vi "Module - Network Stream HMI.vi"(11 "Stop":bool) -> ()   [LabVIEW 2020]
uses:
  Control/State - NS HMI.ctl
  Control/State - eFGV.ctl
  Control/Section.ctl
  <vilib>/dex/Stream Element Allocation Mode.ctl
  <resource>/objmgr/ni.dex.rc
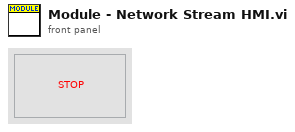
[diagram p1: front panel]
types:
  T1 = cluster{"T_Out":i32, "Event Ref":refnum<event-registration>, "NS Connected?":bool, "NS Endpoint":refnum<k21>, "Stop Main":bool, "NS Setting":cluster{"Timeout":i32, "Buffer Size":i32, "Ip Address":string, "Writer Name":string}}
  T2 = typedef "State - NS HMI.ctl" = enum16{"Init", "Register Event", "Read NS Setting", "Idle", "Create Reader Endpoint", "Check Connection Network Stream", "Read Stream Data", "Destroy NS", "Unregister Event", "Close"}
  T3 = typedef "State - eFGV.ctl" = enum16{"Init", "Read", "Write", "Exit"}
  T4 = enum16{"Timeout", "Buffer Size", "Ip Address", "Writer Name"}
  T5 = typedef "Section.ctl" = enum16{"Software Setup", "Config", "Setup", "Network Stream", "MQTT Client", "Setting", "Sample Interval", "Calibration", "Pre-Ranging", "Overrun", "Static", "Filter", "Properties", "Alarm", "Device", "Logging"}
  T6 = typedef "Stream Element Allocation Mode.ctl" = u32
  T7 = enum32{"invalid app kind", "Development System", "Run Time System", "Student Edition", "Embedded LabVIEW", "Evaluation", "Custom"}
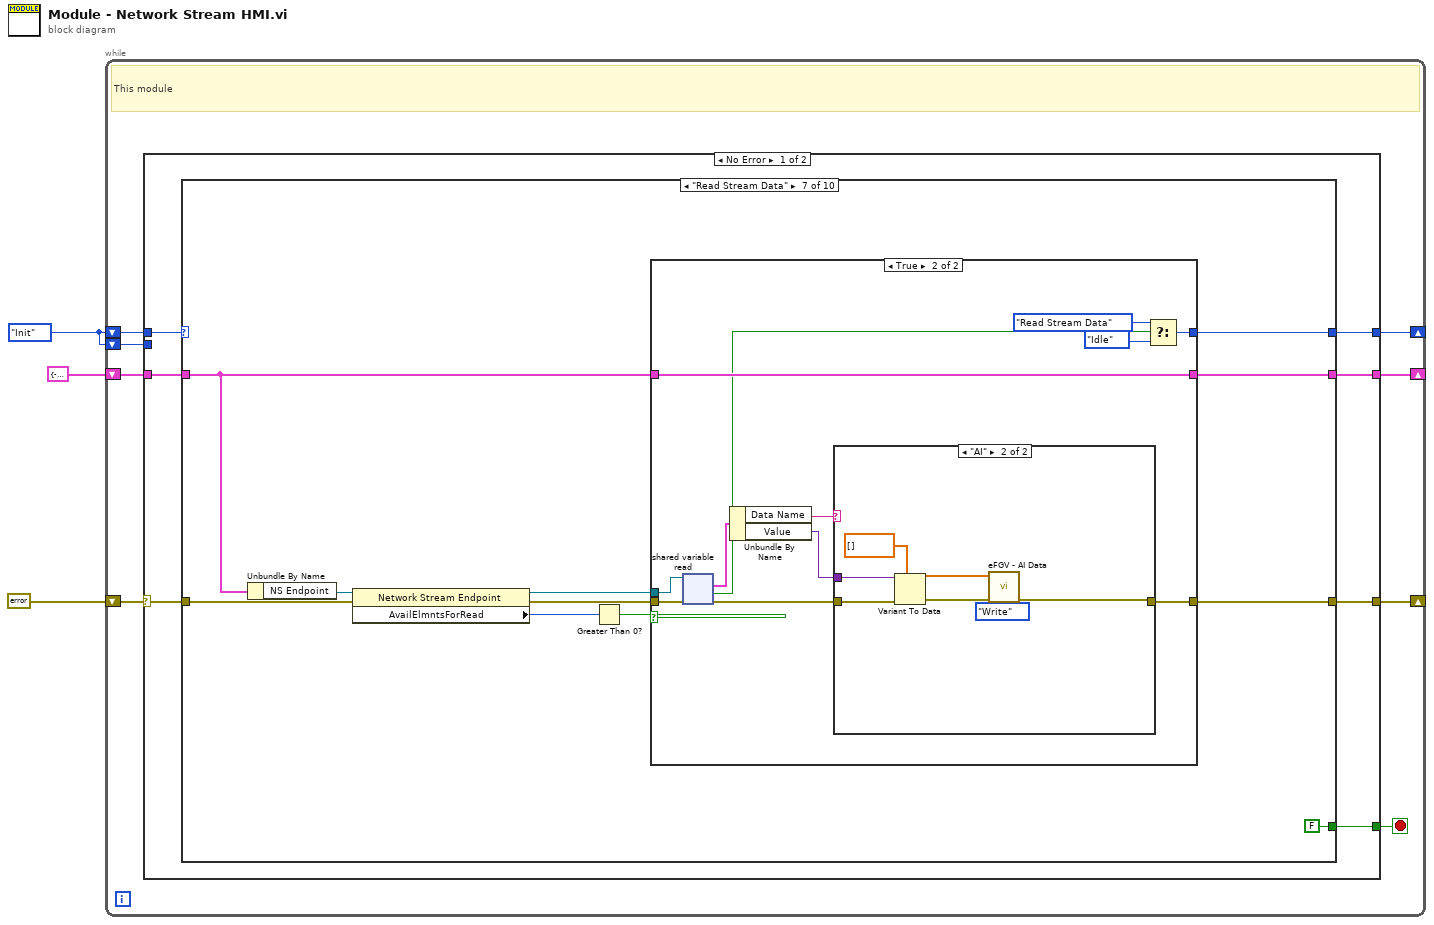
[diagram p0: block diagram]
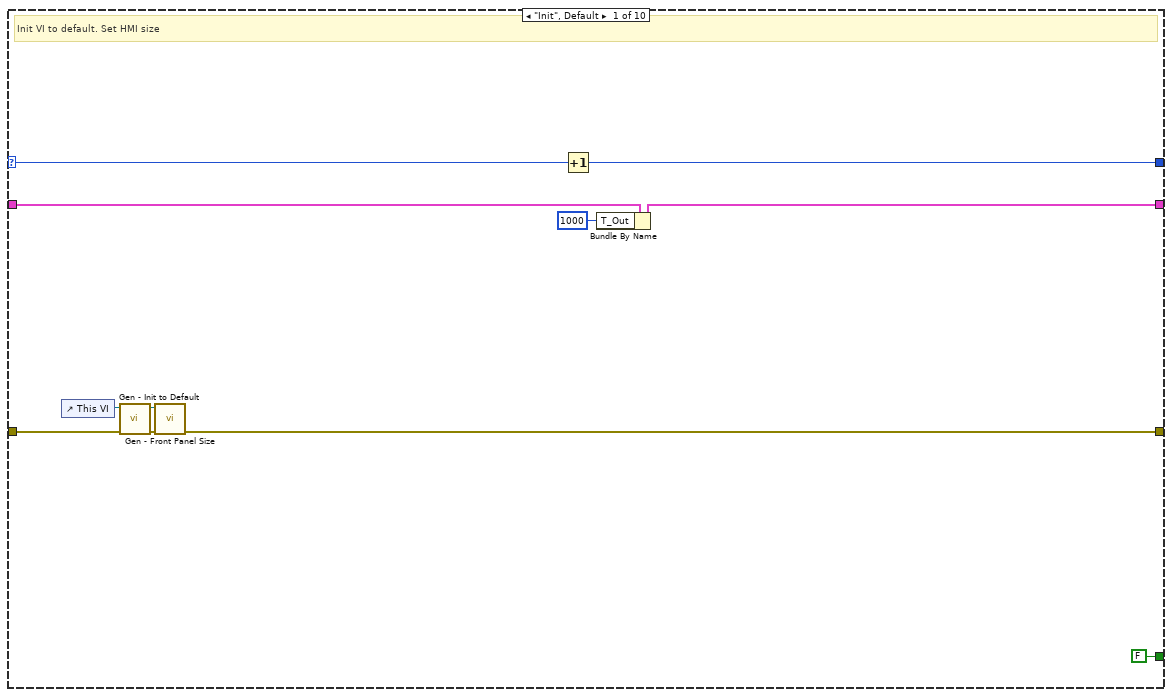
[diagram p2: hidden frame]
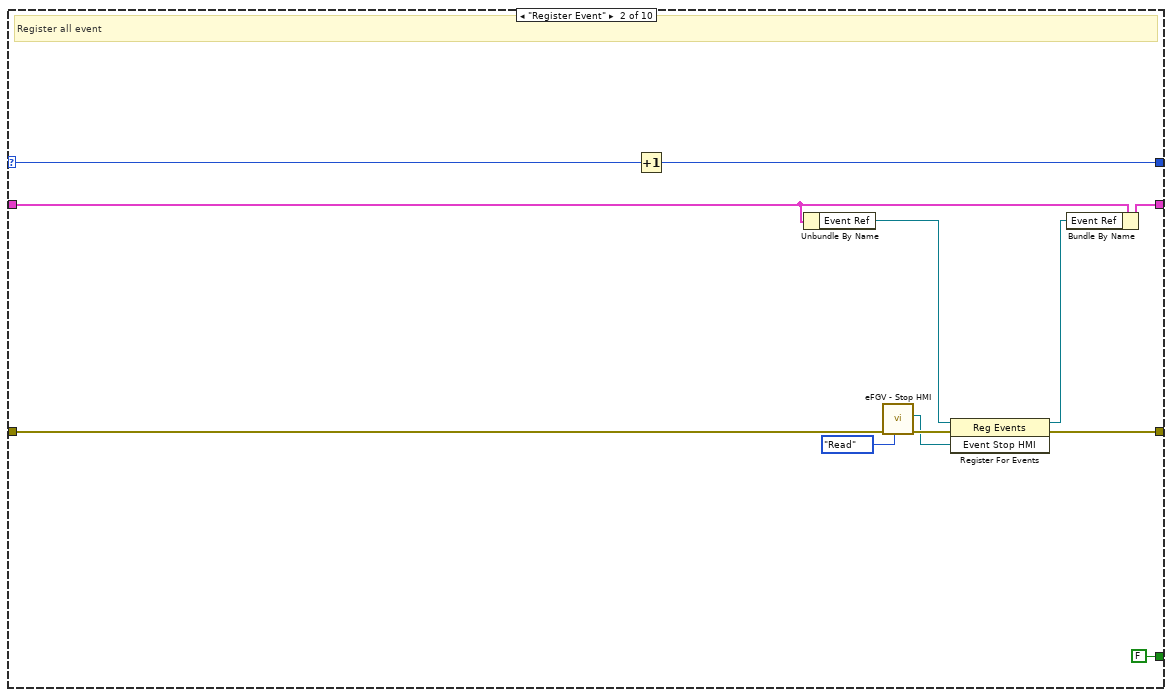
[diagram p3: hidden frame]
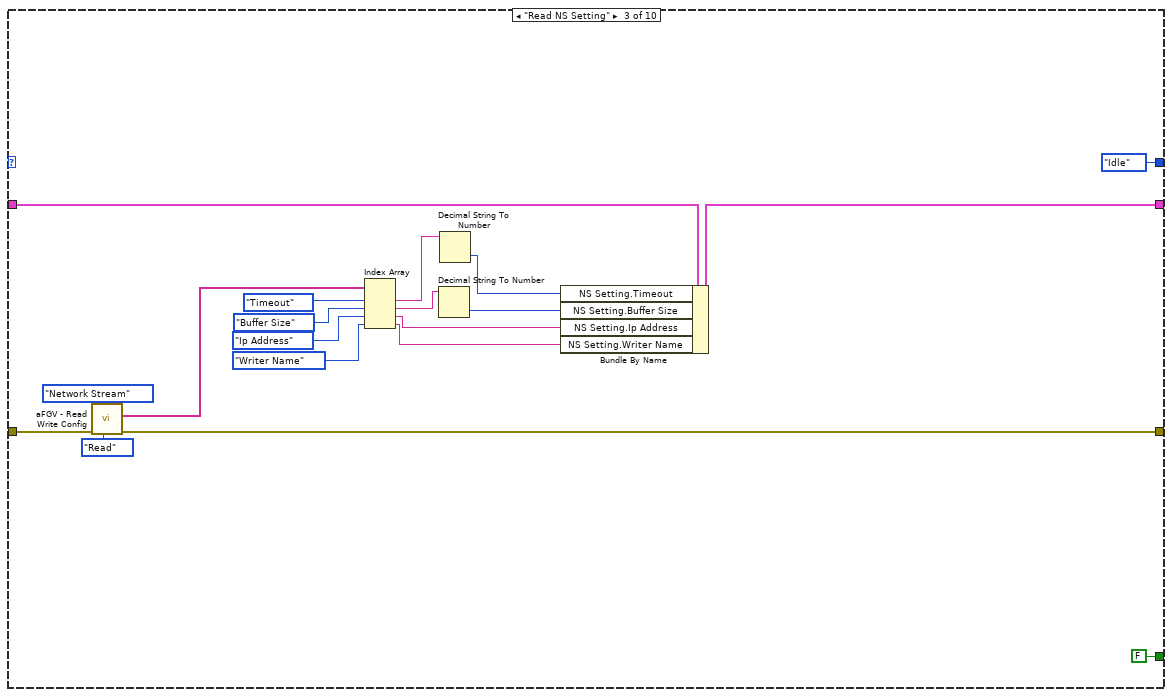
[diagram p4: hidden frame]
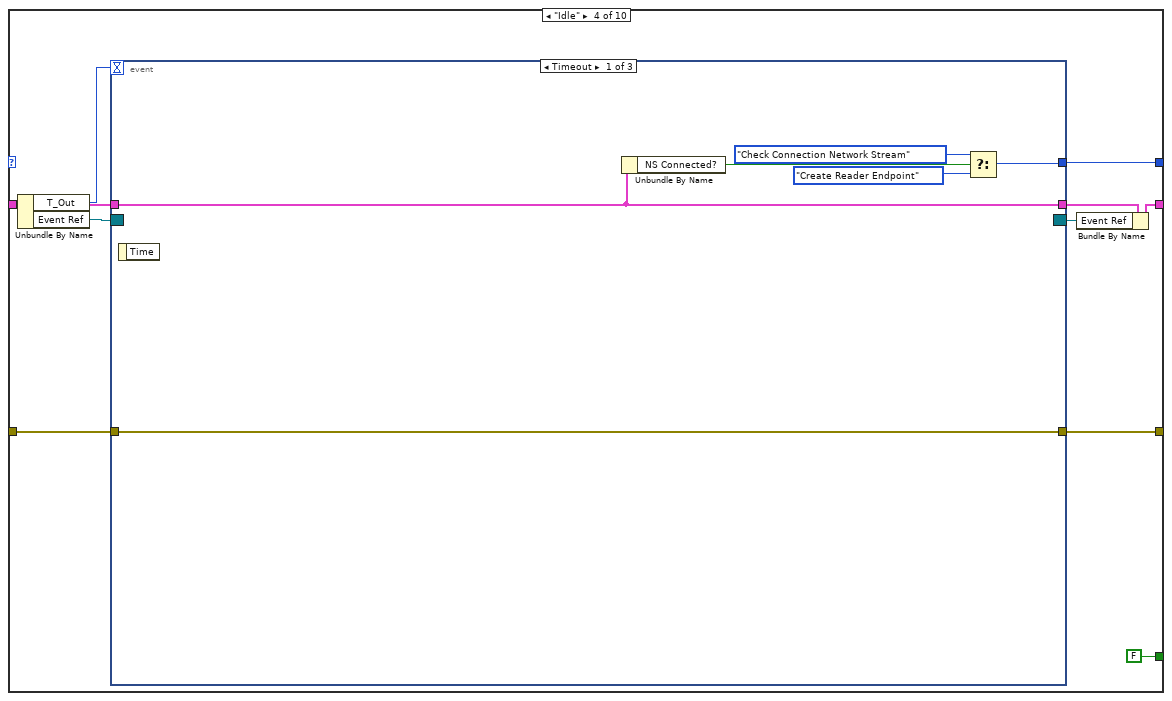
[diagram p5: hidden frame]
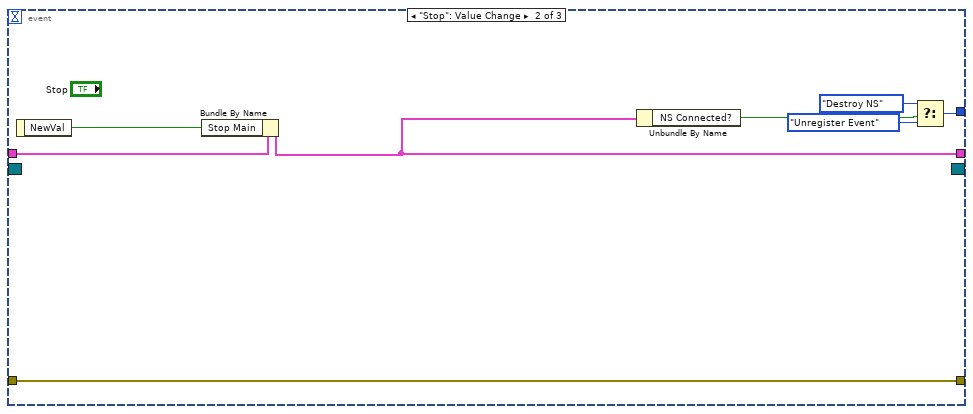
[diagram p6: hidden frame]
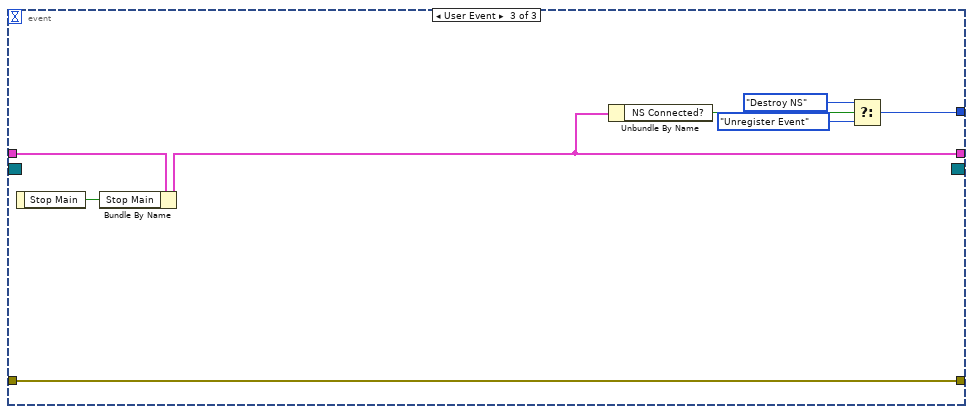
[diagram p7: hidden frame]
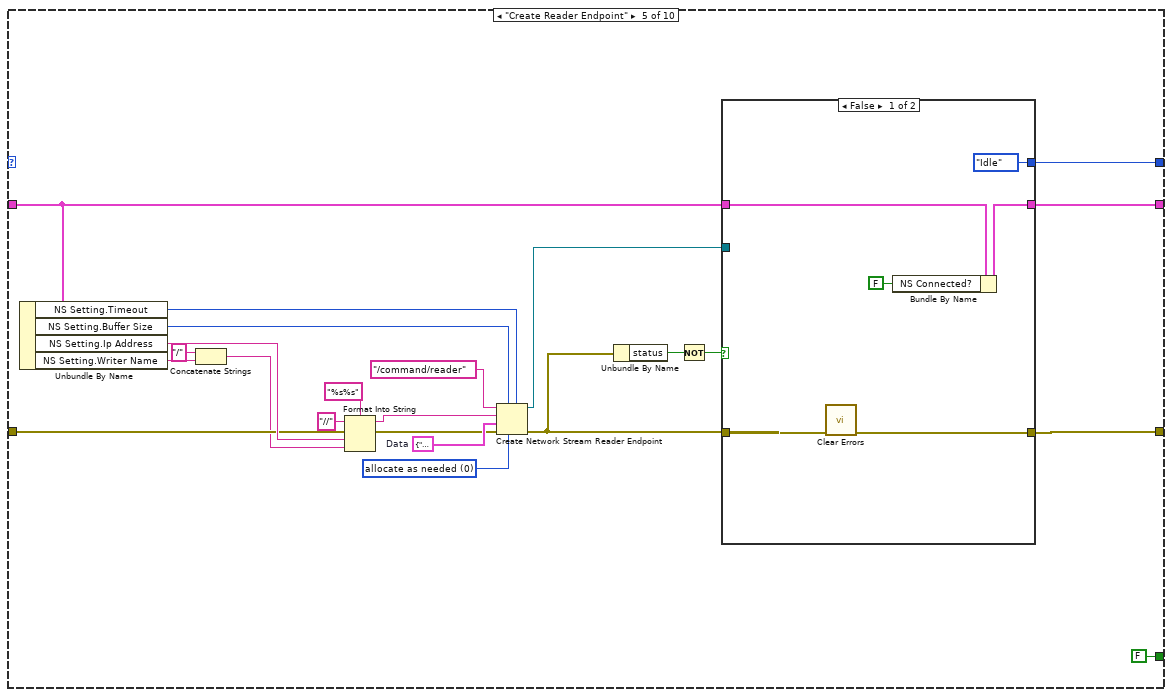
[diagram p8: hidden frame]
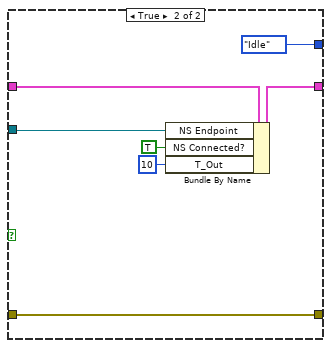
[diagram p9: hidden frame]
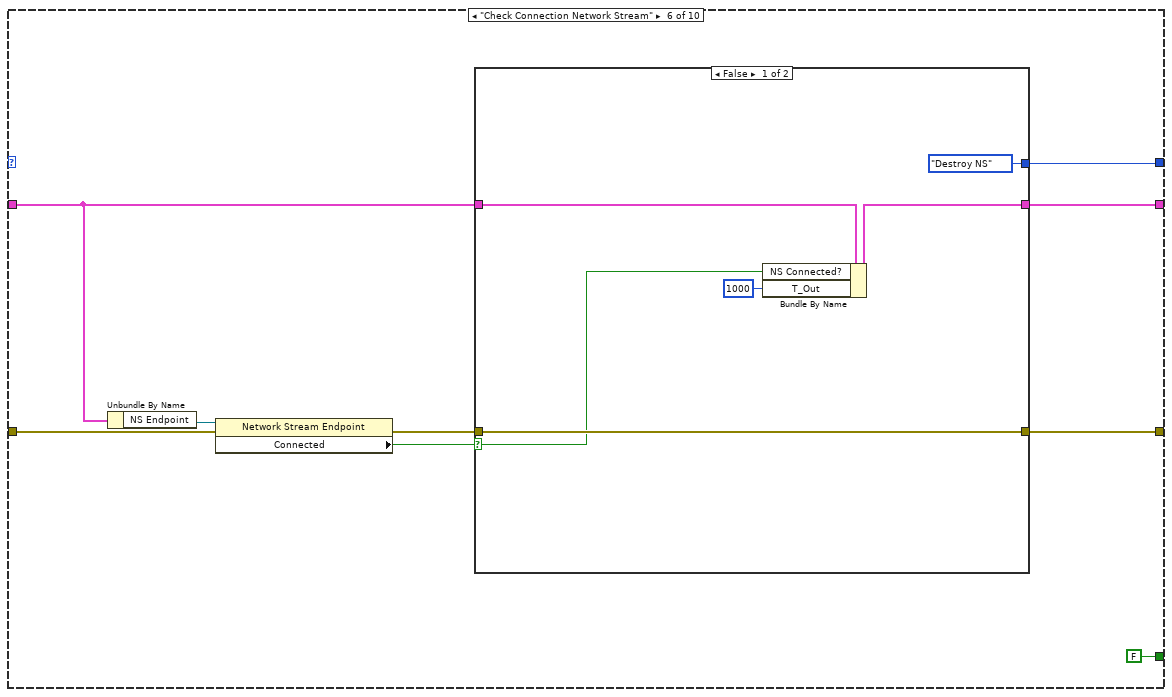
[diagram p10: hidden frame]
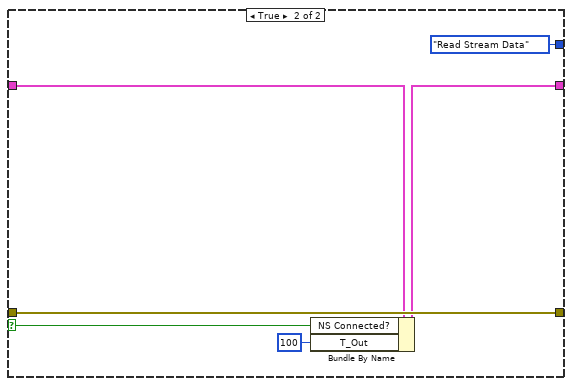
[diagram p11: hidden frame]
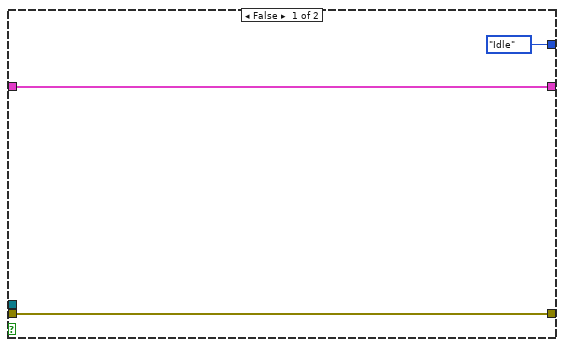
[diagram p12: hidden frame]
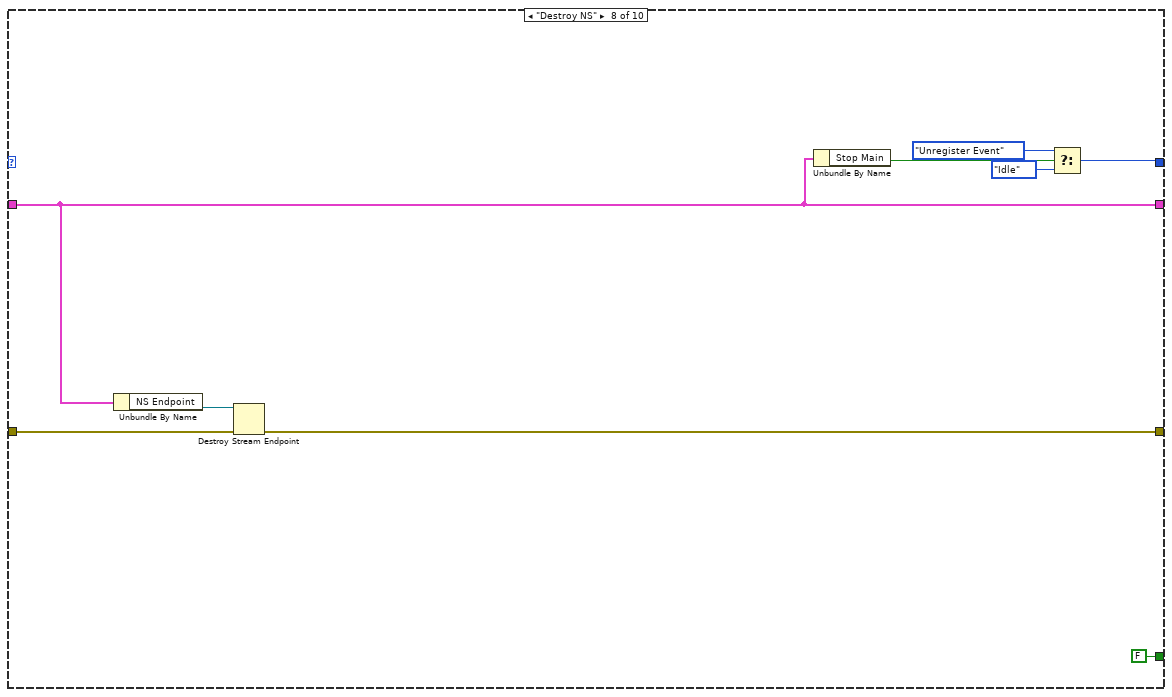
[diagram p14: hidden frame]
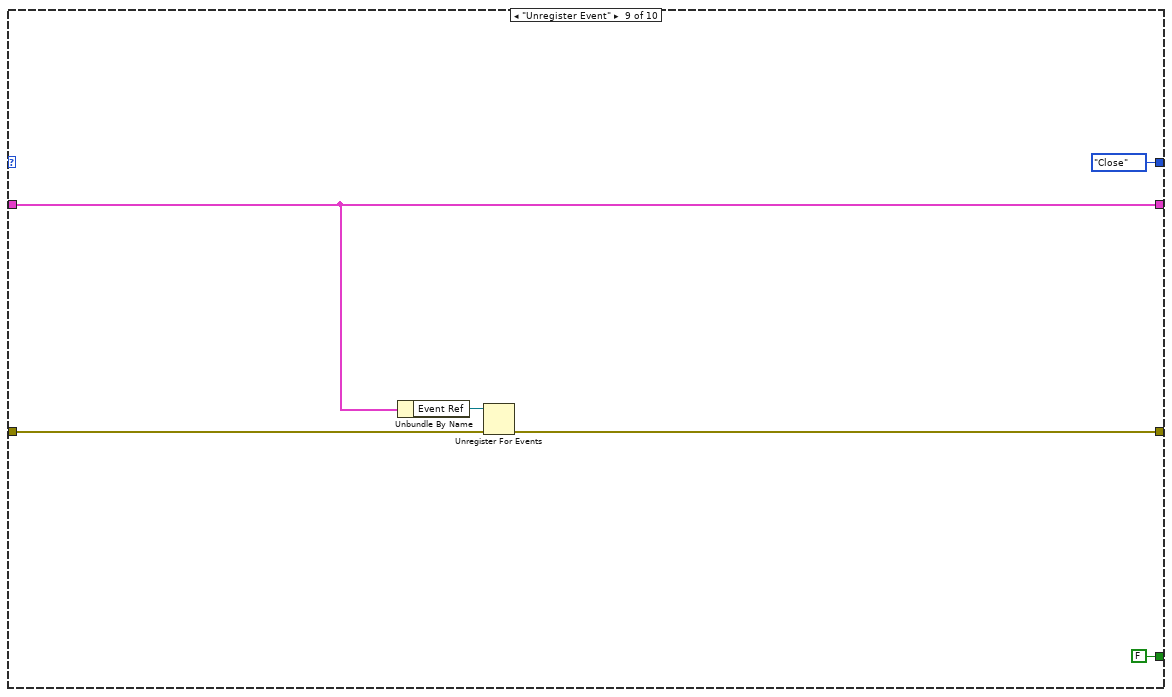
[diagram p15: hidden frame]
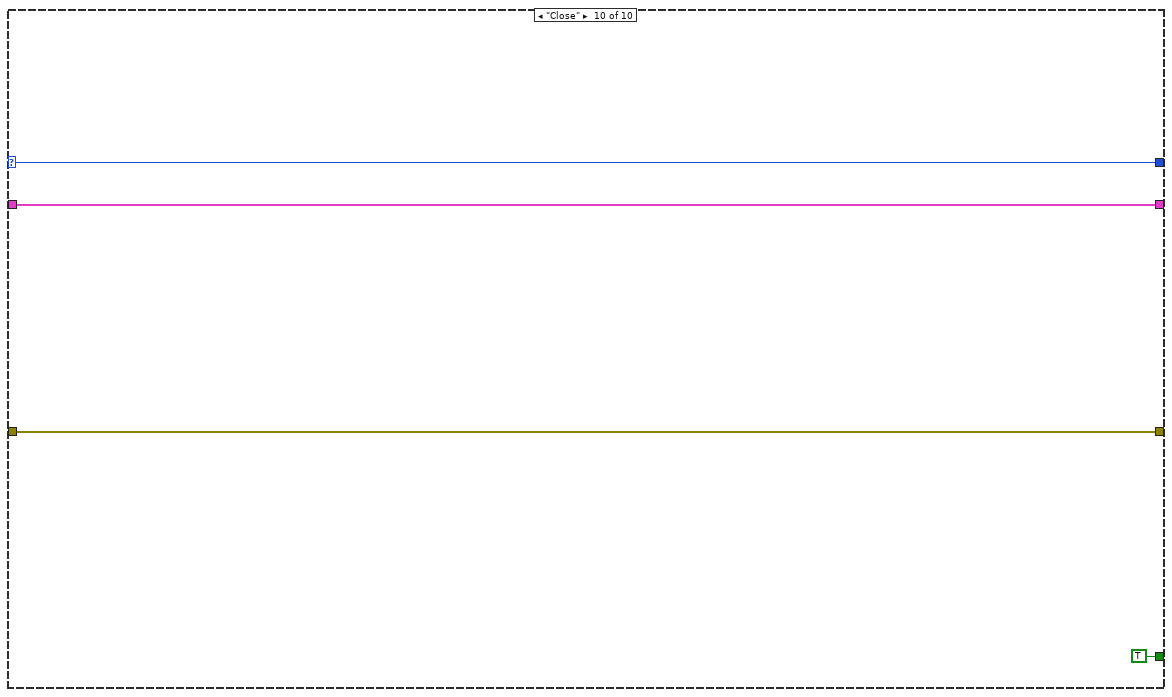
[diagram p16: hidden frame]
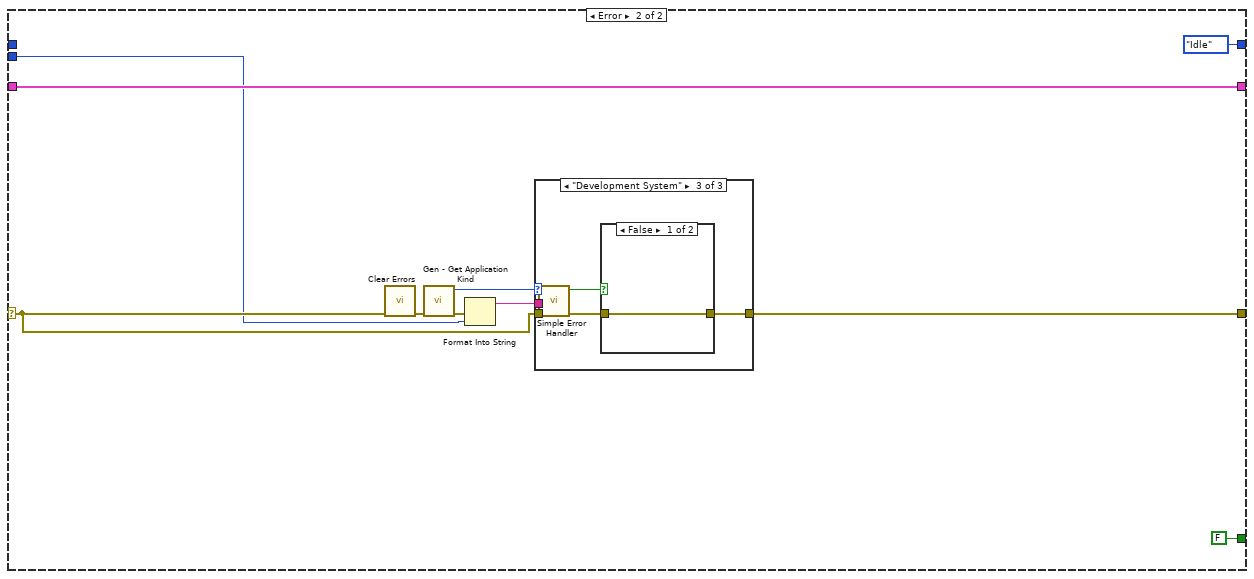
[diagram p17: hidden frame]
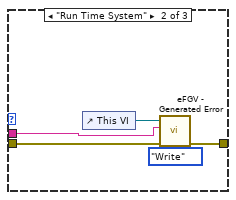
[diagram p19: hidden frame]
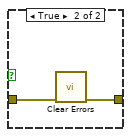
[diagram p20: hidden frame]
diagram:
  w2 = State_-_NS_HMI."Init"
  n1 = while {
    shift-right: [w7] -> _
    shift-left: w2 -> [w9]
    shift-right: [w10] -> _
    shift-left: errorcluster {"status"=FALSE, "code"=0, "source"=""} ("Error In") -> [w11]
    shift-right: [w5] -> _
    shift-left: T1 {"T_Out"=-1, "Event Ref"=refnum, "NS Connected?"=FALSE, "NS Endpoint"="", "Stop Main"=FALSE, "NS Setting"={"Timeout"=0, "Buffer Size"=0, "Ip Address"="", "Writer Name"=""}} -> [w6]
    shift-left: w2 -> [w4]
    stop <- w8 stop-if-true
    # "This module"
    n2 = case shown="No Error" w11 {
      selector: w11 -> [w17 w207]
      tunnel: w9 -> [w16 _]
      tunnel: [w18 w208] -> w10
      tunnel: [w15 FALSE] -> w8
      tunnel: [w14 State_-_NS_HMI."Idle"] -> w7
      tunnel: w6 -> [w13 w211]
      tunnel: [w12 w211] -> w5
      tunnel: w4 -> [_ w204]
      frame No Error {
        n3 = case shown="\"Read Stream Data\"" w16 {
          selector: w16 -> [w24 w37 _ _ _ _ _ _ _ w202]
          tunnel: [w27 w41 w57 w70 w112 w133 w155 w185 w195 w199] -> w18
          tunnel: w17 -> [w29 w39 w58 w69 w99 w137 w160 w192 w196 w199]
          tunnel: [FALSE FALSE FALSE FALSE FALSE FALSE FALSE FALSE FALSE TRUE] -> w15
          tunnel: [w20 w30 State_-_NS_HMI."Idle" w67 w108 w130 w153 w190 State_-_NS_HMI."Close" w202] -> w14
          tunnel: w13 -> [w26 w34 w60 w65 w105 w132 w151 w186 w193 w200]
          tunnel: [w21 w32 w49 w63 w109 w131 w152 w186 w193 w200] -> w12
          frame "Init", Default {
            # "Init VI to default. Set HMI size"
            n4 = control-ref of="This VI"() -> (w23:refnum<vi>)
            n5 = call "Gen - Init to Default.vi"("Error in"=w29, "This VI"=w23) -> ("Error out"=w28:errorcluster, "This VI Copy"=w22:refnum<vi>)  [unwired: 8 in]
            n6 = call "Gen - Front Panel Size.vi"("Error In"=w28, "This VI"=w22) -> ("Error Out"=w27:errorcluster)  [unwired: 9 in]
            n7 = Increment(x=w24) -> (x+1=w20:T2)
            n8 = Bundle By Name(cluster=w26, "T_Out"=1000) -> (w21:T1)
          }
          frame "Register Event" {
            # "Register all event"
            n9 = Increment(x=w37) -> (x+1=w30:T2)
            n10 = Unbundle By Name(w34) -> ("Event Ref"=w33:refnum<event-registration>)
            n11 = call "eFGV - Stop HMI.vi"("Action"=State_-_eFGV."Read", "Error In"=w39) -> ("Error Out"=w40:errorcluster, "Event Stop HMI"=w36:refnum<user-event>)  [unwired: 7 in, 1 out]
            n12 = register-events(reference=w33, error in=w40, w36) -> (reference out=w31:refnum<event-registration>, error out=w41:errorcluster)
            n13 = Bundle By Name(cluster=w34, "Event Ref"=w31) -> (w32:T1)
          }
          frame "Read NS Setting" {
            n14 = call "aFGV - Read Write Config.vi"("State"=enum16{"Read", "Write", "Delete"}."Read", "Section"=Section."Network Stream", "Error In"=w58) -> ("Error Out"=w57:errorcluster, "Data out"=w53:string[])  [unwired: 6 in, 1 out]
            n15 = Index Array(array=w53, index #1=enum16{"Timeout", "Buffer Size", "Ip Address"}."Timeout", index #2=enum16{"Timeout", "Buffer Size", "Ip Address"}."Buffer Size", index #3=T4."Ip Address", index #4=T4."Writer Name") -> (element #1=w47:string, element #2=w46:string, element #3=w44:string, element #4=w43:string)
            n16 = Decimal String To Number(string=w46) -> (number=w45:i32)  [unwired: 2 in, 1 out]
            n17 = Decimal String To Number(string=w47) -> (number=w42:i32)  [unwired: 2 in, 1 out]
            n18 = Bundle By Name(cluster=w60, "NS Setting.Timeout"=w42, "NS Setting.Buffer Size"=w45, "NS Setting.Ip Address"=w44, "NS Setting.Writer Name"=w43) -> (w49:T1)
          }
          frame "Idle" {
            n19 = Unbundle By Name(w65) -> ("T_Out"=w61:i32, "Event Ref"=w64:refnum<event-registration>)
            n20 = event shown="[0] Timeout" {
              selector: w64 -> [_ _ _]
              dyn-events: [_ _ _] -> w62
              timeout: w61 -> [_ _ _]
              tunnel: [w76 w84 w92] -> w70
              tunnel: w69 -> [w76 w84 w92]
              tunnel: [w71 w81 w85] -> w67
              tunnel: [w75 w79 w89] -> w66
              tunnel: w65 -> [w75 w83 w91]
              event Timeout {
                n21 = event-data() -> ()  [unwired: 1 in, 1 out]
                n22 = Unbundle By Name(w75) -> ("NS Connected?"=w74:bool)
                n23 = Select(t=State_-_NS_HMI."Check Connection Network Stream", s=w74, f=State_-_NS_HMI."Create Reader Endpoint") -> (s? t:f=w71:T2)
              }
              event "Stop": Value Change {
                n24 = event-data() -> ("NewVal"=w82:bool)  [unwired: 1 in]
                n25 = Bundle By Name(cluster=w83, "Stop Main"=w82) -> (w79:T1)
                n26 = Unbundle By Name(w79) -> ("NS Connected?"=w78:bool)
                n27 = Select(t=State_-_NS_HMI."Destroy NS" ("f"), s=w78, f=State_-_NS_HMI."Unregister Event") -> (s? t:f=w81:T2)
              }
              event User Event {
                n28 = event-data() -> ("Stop Main"=w90:bool)  [unwired: 1 in]
                n29 = Bundle By Name(cluster=w91, "Stop Main"=w90) -> (w89:T1)
                n30 = Unbundle By Name(w89) -> ("NS Connected?"=w88:bool)
                n31 = Select(t=State_-_NS_HMI."Destroy NS" ("f"), s=w88, f=State_-_NS_HMI."Unregister Event") -> (s? t:f=w85:T2)
              }
            }
            n32 = Bundle By Name(cluster=w66, "Event Ref"=w62) -> (w63:T1)
          }
          frame "Create Reader Endpoint" {
            w106 = T6 0 items=["allocate as needed", "pre-allocate"] ("element allocation mode")
            w107 = cluster{"Data Name":string, "Value":variant} {"Data Name"="", "Value"=variant}  # Data
            n33 = Unbundle By Name(w105) -> ("NS Setting.Timeout"=w104:i32, "NS Setting.Buffer Size"=w103:i32, "NS Setting.Ip Address"=w102:string, "NS Setting.Writer Name"=w97:string)
            n34 = Concatenate Strings("/" ("string"), w97) -> (w96:string)
            n35 = Format Into String(format string="%s%s", initial string="//", error in=w99, w102, w96) -> (resulting string=w100:string, error out=w98:errorcluster)
            n36 = Create Network Stream Reader Endpoint(5:w104, 6:w106, 7:w103, 8:w98, 9:w107, 10:w100, 11:"/command/reader" ("reader url")) -> (0:w115:errorcluster, 3:w110:refnum<k21>)
            n37 = Unbundle By Name(w115) -> ("status"=w114:bool)
            n38 = Not(x=w114) -> (.not. x?=w113:bool)
            n39 = case shown="False" w113 {
              tunnel: w115 -> [w117 w128]
              tunnel: [w116 w128] -> w112
              tunnel: w105 -> [w121 w127]
              tunnel: w110 -> [_ w124]
              tunnel: [w119 w125] -> w109
              tunnel: [State_-_NS_HMI."Idle" State_-_NS_HMI."Idle"] -> w108
              frame False {
                n40 = call <vilib>:"Clear Errors.vi"("error in (no error)"=w117) -> ("error out"=w116:errorcluster)  [unwired: 5 in, 1 out]
                n41 = Bundle By Name(cluster=w121, "NS Connected?"=FALSE) -> (w119:T1)
              }
              frame True {
                n42 = Bundle By Name(cluster=w127, "NS Endpoint"=w124, "NS Connected?"=TRUE, "T_Out"=10) -> (w125:T1)
              }
            }
          }
          frame "Check Connection Network Stream" {
            n43 = Unbundle By Name(w132) -> ("NS Endpoint"=w135:refnum<k21>)
            n44 = property class="Network Stream Endpoint"(reference=w135, error in=w137) -> (error out=w134:errorcluster, "Connected"=w129:bool)  [unwired: 1 out]
            n45 = case shown="False" w129 {
              selector: w129 -> [w139 w145]
              tunnel: w134 -> [w142 w149]
              tunnel: [w142 w149] -> w133
              tunnel: w132 -> [w143 w148]
              tunnel: [w140 w146] -> w131
              tunnel: [State_-_NS_HMI."Destroy NS" State_-_NS_HMI."Read Stream Data"] -> w130
              frame False {
                n46 = Bundle By Name(cluster=w143, "NS Connected?"=w139, "T_Out"=1000) -> (w140:T1)
              }
              frame True {
                n47 = Bundle By Name(cluster=w148, "NS Connected?"=w145, "T_Out"=100) -> (w146:T1)
              }
            }
          }
          frame "Read Stream Data" {
            n48 = Unbundle By Name(w151) -> ("NS Endpoint"=w159:refnum<k21>)
            n49 = property class="Network Stream Endpoint"(reference=w159, error in=w160) -> (reference out=w150:refnum<k21>, error out=w156:errorcluster, "AvailElmntsForRead"=w158:i32)
            n50 = Greater Than 0?(x=w158) -> (x > 0?=w154:bool)
            n51 = case shown="True" w154 {
              tunnel: w156 -> [w163 w173]
              tunnel: [w163 w174] -> w155
              tunnel: [State_-_NS_HMI."Idle" w167] -> w153
              tunnel: [w161 w175] -> w152
              tunnel: w151 -> [w161 w175]
              tunnel: w150 -> [_ w171]
              frame False {
              }
              frame True {
                n52 = shared-variable-read(w171, w173) -> (w172:errorcluster, w164:bool, w170:cluster{"Data Name":string, "Value":variant})  [unwired: 1 in, 1 out]
                n53 = Unbundle By Name(w170) -> ("Data Name"=w169:string, "Value"=w168:variant)
                n54 = case shown="\"AI\"" w169 {
                  tunnel: w172 -> [w176 w183]
                  tunnel: [w176 w179] -> w174
                  tunnel: w168 -> [_ w182]
                  frame Default {
                  }
                  frame "AI" {
                    n55 = Variant To Data(error in=w183, type=sgl[] [] ("Event AI Calibrated"), Variant=w182) -> (data=w177:sgl[], error out=w180:errorcluster)
                    n56 = call "eFGV - AI Data.vi"("States"=State_-_eFGV."Write", "Error In"=w180, "Event AI Data"=w177) -> ("Error Out"=w179:errorcluster)  [unwired: 7 in, 1 out]
                  }
                }
                n57 = Select(t=State_-_NS_HMI."Read Stream Data", s=w164, f=State_-_NS_HMI."Idle") -> (s? t:f=w167:T2)
              }
            }
          }
          frame "Destroy NS" {
            n58 = Unbundle By Name(w186) -> ("NS Endpoint"=w184:refnum<k21>)
            n59 = Destroy Stream Endpoint(8:w192, 11:w184) -> (0:w185:errorcluster)
            n60 = Unbundle By Name(w186) -> ("Stop Main"=w191:bool)
            n61 = Select(t=State_-_NS_HMI."Unregister Event", s=w191, f=State_-_NS_HMI."Idle") -> (s? t:f=w190:T2)
          }
          frame "Unregister Event" {
            n62 = Unbundle By Name(w193) -> ("Event Ref"=w197:refnum<event-registration>)
            n63 = Unregister For Events(event registration refnum=w197, error in=w196) -> (error out=w195:errorcluster)
          }
          frame "Close" {
          }
        }
      }
      frame Error {
        n64 = call <vilib>:"Clear Errors.vi"("error in (no error)"=w207) -> ("error out"=w210:errorcluster)  [unwired: 5 in, 1 out]
        n65 = call "Gen - Get Application Kind.vi"("Error In"=w210) -> ("Error Out"=w206:errorcluster, "Application:Kind"=w209:T7)  [unwired: 9 in]
        n66 = Format Into String(error in=w206, w204) -> (resulting string=w205:string)  [unwired: 2 in, 1 out]
        n67 = case shown="\"Development System\"" w209 {
          tunnel: [w213 w218 w222] -> w208
          tunnel: w207 -> [w213 w215 w220]
          tunnel: w205 -> [_ w214 _]
          frame "invalid app kind", Default {
          }
          frame "Run Time System" {
            n68 = control-ref of="This VI"() -> (w216:refnum<vi>)
            n69 = call "eFGV - Generated Error.vi"("eFGV States"=State_-_eFGV."Write", "Error In"=w215, "State"=w214, "This VI"=w216) -> ("Error Out"=w218:errorcluster)  [unwired: 6 in, 1 out]
          }
          frame "Development System" {
            n70 = call <vilib>:"Simple Error Handler.vi"("error in (no error)"=w220) -> ("error?"=w219:bool, "error out"=w221:errorcluster)  [unwired: 4 in, 3 out]
            n71 = case shown="False" w219 {
              tunnel: [w223 w225] -> w222
              tunnel: w221 -> [w223 w224]
              frame False {
              }
              frame True {
                n72 = call <vilib>:"Clear Errors.vi"("error in (no error)"=w224) -> ("error out"=w225:errorcluster)  [unwired: 5 in, 1 out]
              }
            }
          }
        }
      }
    }
  }
